vi "Module to Generate Flood of Logs.vi"(7 "Name (\"\" to Use Uuid)":string="CSM-Module") -> ()   [LabVIEW 2017, in "Global Log Handling Capability Example.lvlib"]
doc: "------------- lvcsm -------------\n[CSMStates]\nItem 0 = \"Idle\"\nItem 1 = \"CSM Documentation\"\nItem 2 = \"VI Reference\"\nItem 3 = \"Error Handler\"\nItem 4 = \"Critical Error\"\nItem 5 = \"Target Timeout Error\"\nItem 6 = \"Target Error\"\nItem 7 = \"Async Response\"\nItem 8 = \"Response\"\nItem 9 = \"Async Message Posted\"\nItem 10 = \"Initialize Core Data\"\nItem 11 = \"Exit\"\nItem 12 = \"Data: Initialize\"\nItem 13 = \"Data: Update Indicators\"\nItem 14 = \"Data: Cleanup\"\nItem 15 = \"Macro: Initialize\"\nItem 16 = \"Macro: Exit\"\nItem 17 = \"API: API1\"\nItem 18 = \"API: API2\"\nItem 19 = \"Action: Start\"\nItem 20 = \"Action: action2\"\n\n[CSMStatus]\nItem 0 = \"Error Occurred@Error Handler\""
uses:
  Global Log Handling Capability Example.lvlib
  user.lib/_NEVSTOP/Communicable State Machine(CSM)/AdvanceAPI/CSM - Revert Arguments-Safe String.vi
  user.lib/_NEVSTOP/Communicable State Machine(CSM)/AdvanceAPI/CSM - Make String Arguments Safe.vi
  user.lib/_NEVSTOP/Communicable State Machine(CSM)/AdvanceAPI/CSM - Break Down Multiple States String.vi
  user.lib/_NEVSTOP/Communicable State Machine(CSM)/AdvanceAPI/CSM - Compact Multiple States.vi
  user.lib/_NEVSTOP/Communicable State Machine(CSM)/AdvanceAPI/CSM - Keywords.vi
  user.lib/_NEVSTOP/Communicable State Machine(CSM)/_Shared/Trim Single-line Text.vi
  user.lib/_NEVSTOP/Communicable State Machine(CSM)/Communicable State Machine.lvlib
  user.lib/_NEVSTOP/Communicable State Machine(CSM)/addons/Loop-Support/CSM Loop Support.lvlib
panel:
  in  "Exit":bool
  out "Error Occurred":errorcluster
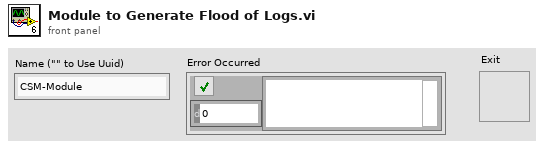
[diagram p1: front panel]
types:
  T1 = enum32{"Invalid", "Standard", "Closed", "Hidden", "Minimized", "Maximized"}
  T2 = enum32{"invalid app kind", "Development System", "Run Time System", "Student Edition", "Embedded LabVIEW", "Evaluation", "Custom"}
  T3 = typedef "Communicable State Machine.lvlib/_CSM_Response Source Message.ctl" = cluster{"‘State":string, "’Arguments":string, "’Error":errorcluster}
  T4 = cluster{"Current VI Reference":refnum<vi>, "Close Panel on Exit?":bool}
  T5 = cluster{"Core":cluster{"Current VI Reference":refnum<vi>, "Close Panel on Exit?":bool}, "Your Boolean data":bool, "Your string data":string}
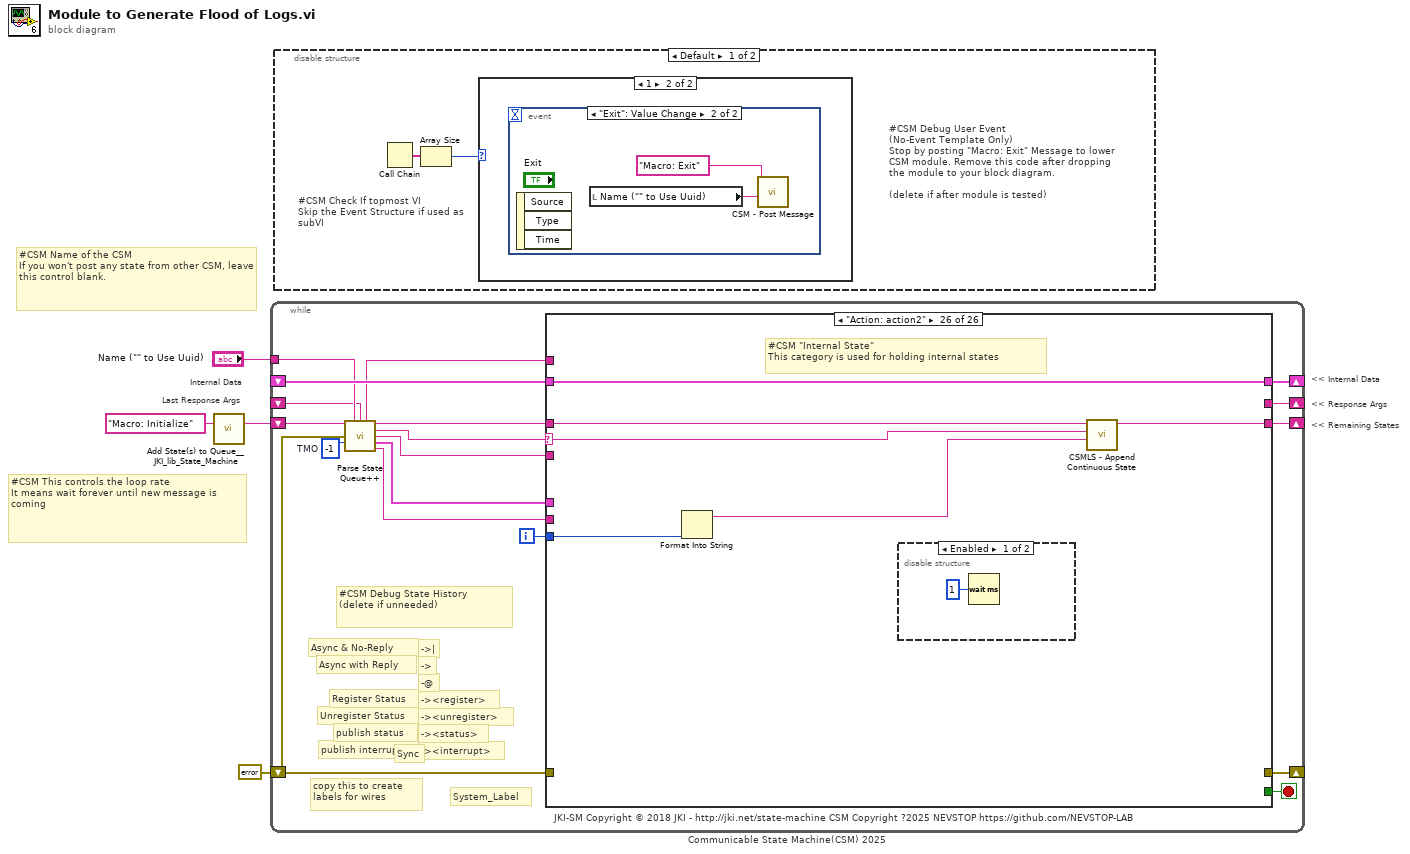
[diagram p0: block diagram]
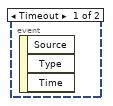
[diagram p3: hidden frame]
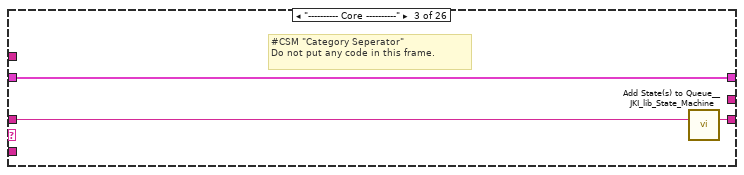
[diagram p7: hidden frame]
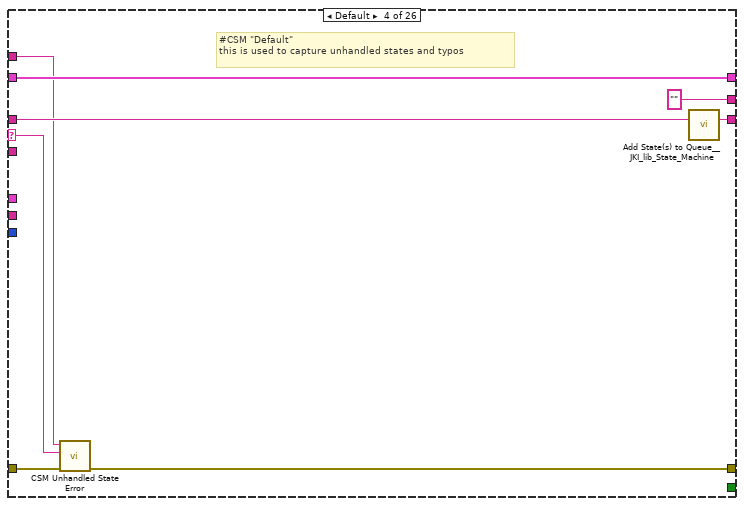
[diagram p8: hidden frame]
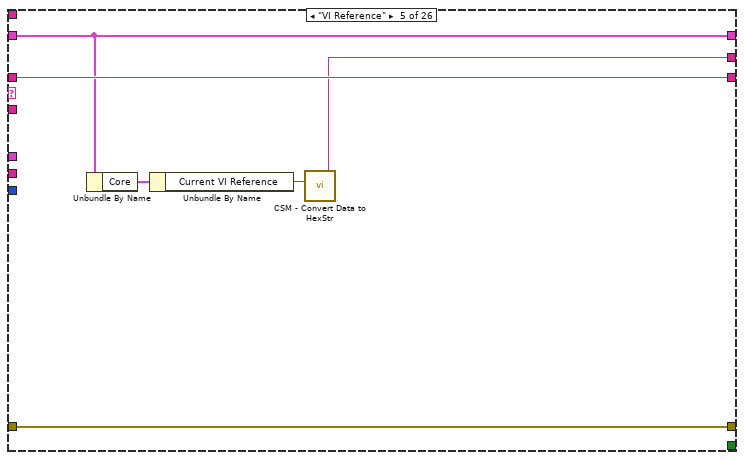
[diagram p9: hidden frame]
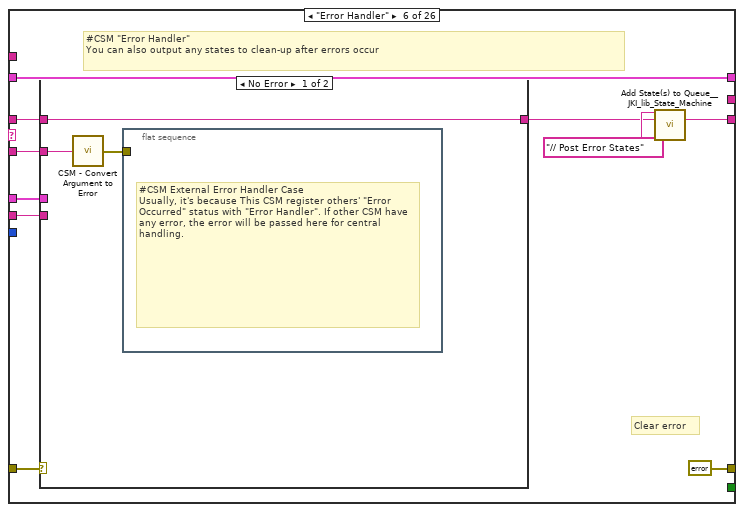
[diagram p10: hidden frame]
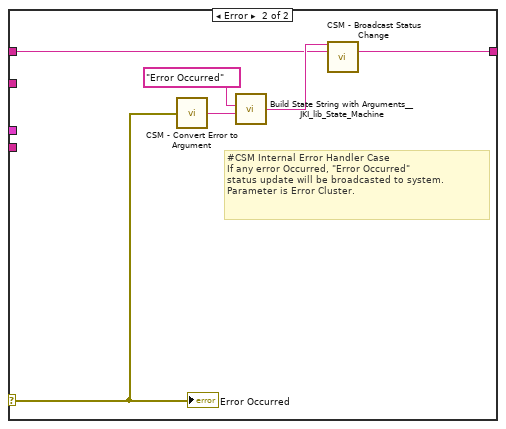
[diagram p11: hidden frame]
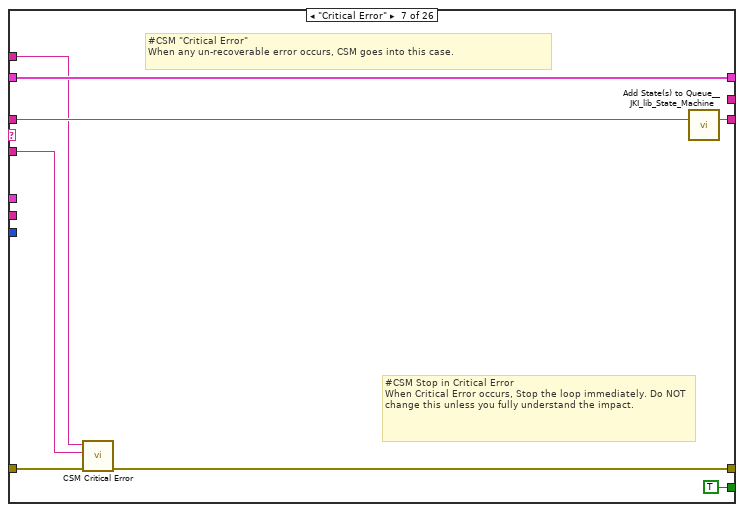
[diagram p12: hidden frame]
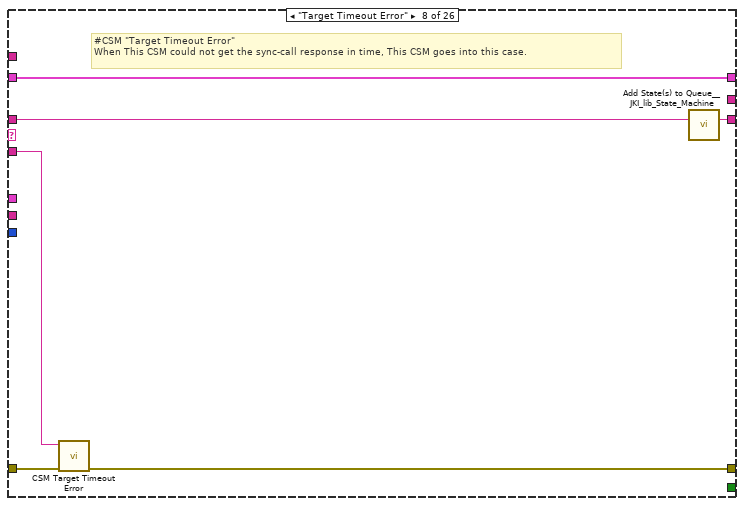
[diagram p13: hidden frame]
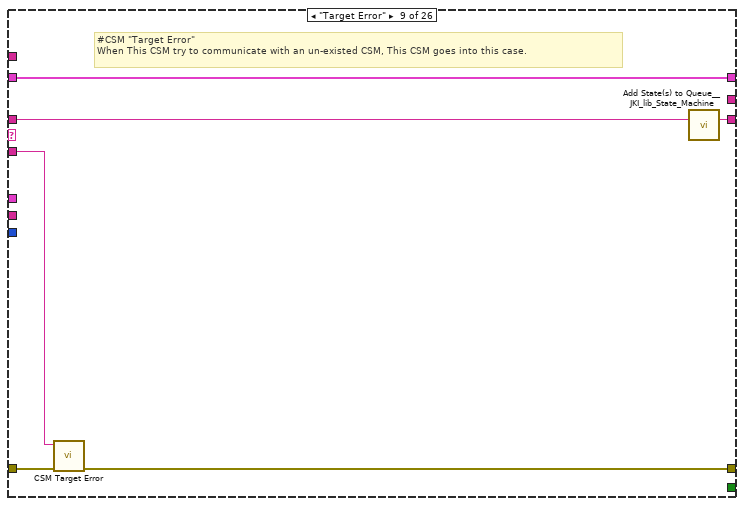
[diagram p14: hidden frame]
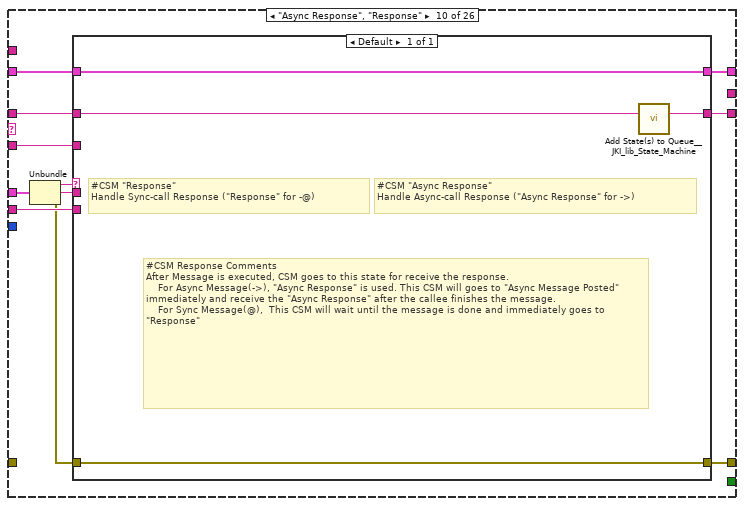
[diagram p15: hidden frame]
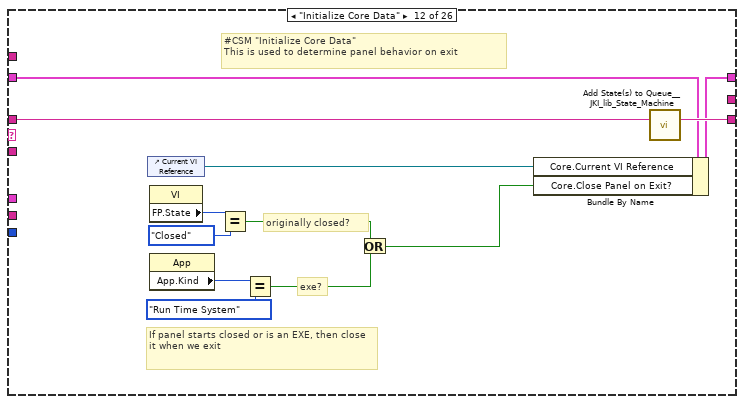
[diagram p17: hidden frame]
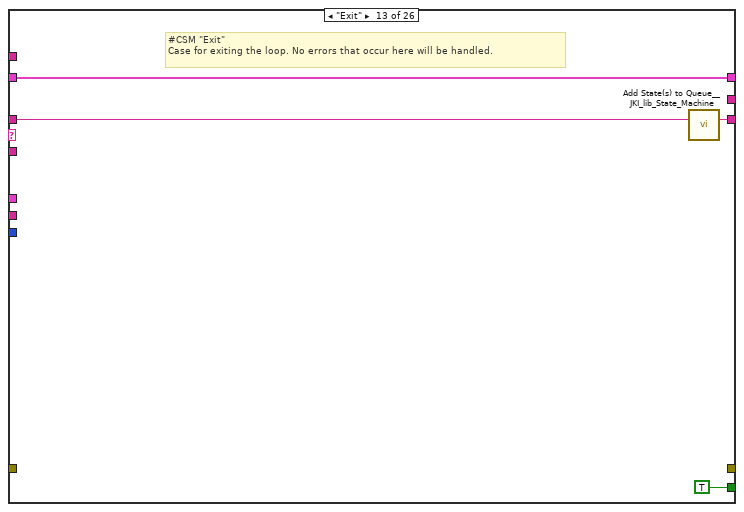
[diagram p18: hidden frame]
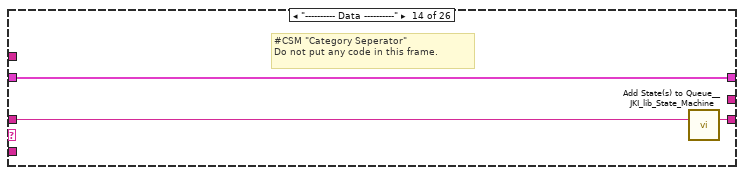
[diagram p19: hidden frame]
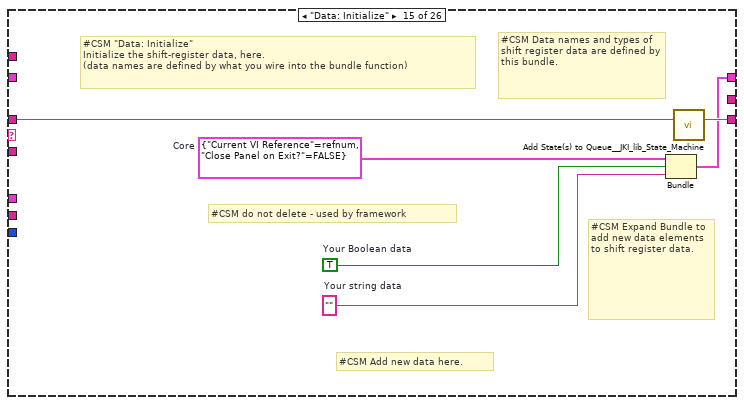
[diagram p20: hidden frame]
diagram:
  # "Last Response Args"
  # "Internal Data"
  # "#CSM Name of the CSM\nIf you won't post any state from other CSM, leave this control blank."
  # "#CSM This controls the loop rate\nIt means wait forever until new message is coming"
  # "<< Internal Data"
  # "<< Response Args"
  # "<< Remaining States"
  n1 = call <vilib>:"Add State(s) to Queue__JKI_lib_State_Machine.vi"("State(s) in (\"\")"="Macro: Initialize" ("Init State(\"Macro: Initialize\")")) -> ("States Out"=w4:string)  [unwired: 14 in]
  n2 = while "Communicable State Machine(CSM) 2025" {
    shift-right: [w17] -> _
    shift-left: _ -> [w16]
    shift-right: [w20] -> _
    shift-left: errorcluster {"status"=FALSE, "code"=0, "source"=""} ("error out") -> [w6]
    shift-right: [w19] -> _
    shift-left: w4 -> [w21]
    tunnel: "Name (\"\" to Use Uuid)" -> [w13]
    shift-right: [w14] -> _
    shift-left: _ -> [w8]
    i -> [w5]
    stop <- w18 stop-if-true
    w15 = -1  # TMO
    # "#CSM Debug State History\n(delete if unneeded)"
    # "-><interrupt>"
    # "-><status>"
    # "-><unregister>"
    # "-><register>"
    # "-@"
    # "->"
    # "->|"
    # "publish interrupt"
    # "publish status"
    # "Unregister Status"
    # "Register Status"
    # "Sync"
    # "Async with Reply"
    # "Async & No-Reply"
    # "JKI-SM Copyright © 2018 JKI - http://jki.net/state-machine CSM Copyright ?2025 NEVSTOP https://github.com/NEVSTOP-LAB"
    # "copy this to create labels for wires"
    # "System_Label"
    n3 = call "Parse State Queue++.vi"("State Queue"=w21, "Name (\"\" to Use UUID)"=w13, "Response Arguments"=w8, "Previous Error"=w6, "Dequeue (1 ms)"=w15) -> ("Name Used"=w7:string, "Remaining States"=w22:string, "Current State"=w9:string, "Arguments"=w10:string, "Additional Information"=w11:T3, "Source CSM"=w12:string)  [unwired: 5 in]
    n4 = case shown="\"Action: action2\"" w9 {
      selector: w9 -> [_ _ _ w33 _ _ _ _ _ _ _ _ _ _ _ _ _ _ _ _ _ _ _ _ _ w166]
      tunnel: w22 -> [w23 w26 w29 w37 w42 w47 w70 w76 w82 w92 w99 w111 w115 w118 w124 w126 w132 w135 w139 w145 w147 w150 w154 w159 w163 w167]
      tunnel: w10 -> [_ _ _ _ _ w46 w66 w73 w79 w86 _ _ _ _ _ _ _ _ _ _ _ _ w152 _ _ _]
      tunnel: w16 -> [w24 w25 w27 w35 w41 w52 w68 w74 w80 w90 w98 w105 w113 w116 _ w125 w127 w133 w137 w143 w146 w149 w153 w157 w161 w168]
      tunnel: [_ _ _ w30 w43 errorcluster {"status"=FALSE, "code"=0, "source"=""} ("error out") w63 w71 w77 w93 _ _ _ _ _ _ w128 _ _ _ _ _ _ _ _ _] -> w20
      tunnel: w6 -> [_ _ _ w31 w43 w50 w64 w72 w78 _ _ _ _ _ _ _ w129 _ _ _ _ _ _ _ _ _]
      tunnel: [w23 w26 w28 w36 w42 w48 w69 w75 w81 w91 w99 w110 w114 w117 w123 w126 w131 w134 w138 w144 w147 w150 w154 w158 w162 w169] -> w19
      tunnel: [_ _ _ _ _ _ TRUE _ _ _ _ _ TRUE _ _ _ _ _ _ _ _ _ _ _ _ _] -> w18
      tunnel: [w24 w25 w27 w35 w41 w52 w68 w74 w80 w89 w98 w109 w113 w116 w122 w125 w127 w133 w137 w143 w146 w149 w153 w157 w161 w168] -> w17
      tunnel: w12 -> [_ _ _ _ _ w45 _ _ _ w87 _ _ _ _ _ _ _ _ _ _ _ _ _ _ _ _]
      tunnel: w11 -> [_ _ _ _ _ w44 _ _ _ w88 _ _ _ _ _ _ _ _ _ _ _ _ _ _ _ _]
      tunnel: [_ _ _ "" w38 _ _ _ _ _ _ _ _ _ _ _ _ _ _ _ _ "API1 Response" w151 _ _ _] -> w14
      tunnel: w7 -> [_ _ _ w32 _ _ w65 _ _ _ _ _ _ _ _ _ _ _ _ _ _ _ _ _ _ _]
      tunnel: w5 -> [_ _ _ _ _ _ _ _ _ _ _ _ _ _ _ _ _ _ _ _ _ _ _ _ _ w165]
      frame "", "Idle" {
        # "#CSM \"Idle/Event Handler\"\nexecutes when the state queue is empty"
      }
      frame "CSM Documentation" {
        # "#CSM State Syntax\n\n// Comment line, all text to the right of “//” will be ignored\n// Local Message Example\nDoSth: DoA >> Arguments\n\n// Sync Call Example\nAPI: xxxx >> Arguments -@ TargetModule\n\n// Async Call Example\nAPI: xxxx >> Arguments -> TargetModule\n\n// Async Call without Reply Example\nAPI: xxxx >> Arguments ->| TargetModule\n\n// Broadcast normal status:\nStatus >> StatusArguments  -><status>\n\n// Broadcast Interrupt status:\nInterrupt >> StatusArguments  -><interrupt>\n\n// Register Source Module's status to Handler Module\nStatus@Source Module >> Handler Module@Handler Module -><register>\n\n// Unegister Source Module's status\nStatus@Source Module >> Handler Module -><unregister>"
        # "#CSM README FIRST\n\nCommunicable State Machine(CSM) is a LabVIEW application framework that builds upon JKI State Machine(JKISM). It follows the pattern of JKISM and extends the keywords to describe message communication between modules, including concepts such as Sync-Message, Async-Message, Subscription/Unsubscription of status - essential elements for creating reusable code modules. For more information, please visit the CSM wiki: https://nevstop-lab.github.io/CSM-Wiki/\n\nFor instructions on JKI State Machine, visit: \n    http://jki.net/state-machine/\nFor information about CSM, visit: \n    https://github.com/NEVSTOP-LAB"
        # "#CSM \"Documentation\"\nCase for holding CSM Documenation"
      }
      frame "---------- Core ----------" {
        # "#CSM \"Category Seperator\"\nDo not put any code in this frame."
        n5 = call <vilib>:"Add State(s) to Queue__JKI_lib_State_Machine.vi"("State(s) in (\"\")"=w29) -> ("States Out"=w28:string)  [unwired: 14 in]
      }
      frame Default {
        # "#CSM \"Default\"\nthis is used to capture unhandled states and typos"
        n6 = call "CSM Unhandled State Error.vi"("error in (no error)"=w31, "Undefined State"=w33, "CSM Name"=w32) -> ("error out"=w30:errorcluster)  [unwired: 8 in]
        n7 = call <vilib>:"Add State(s) to Queue__JKI_lib_State_Machine.vi"("State(s) in (\"\")"=w37) -> ("States Out"=w36:string)  [unwired: 14 in]
      }
      frame "VI Reference" {
        n8 = Unbundle By Name(w41) -> ("Core"=w40:T4)
        n9 = Unbundle By Name(w40) -> ("Current VI Reference"=w39:refnum<vi>)
        n10 = call "CSM - Convert Data to HexStr.vi"("Variant"=w39) -> ("HEX String (0-9,A-F)"=w38:string)  [unwired: 8 in]
      }
      frame "Error Handler" {
        # "#CSM \"Error Handler\"\nYou can also output any states to clean-up after errors occur"
        # "Clear error"
        n11 = case shown="No Error" w50 {
          selector: w50 -> [_ w57]
          tunnel: [w56 w59] -> w49
          tunnel: w47 -> [w56 w58]
          tunnel: w46 -> [w55 _]
          tunnel: w45 -> [_ _]
          tunnel: w44 -> [_ _]
          frame No Error {
            n12 = call "CSM - Convert Argument to Error.vi"("Argument"=w55) -> ("Error"=w54:errorcluster)  [unwired: 4 in]
            n13 = flat-sequence {
              tunnel: w54 -> [_]
              frame #0 {
                # "#CSM External Error Handler Case\nUsually, it's because This CSM register others' \"Error Occurred\" status with \"Error Handler\". If other CSM have any error, the error will be passed here for central handling."
              }
            }
          }
          frame Error {
            # "#CSM Internal Error Handler Case \nIf any error Occurred, \"Error Occurred\" \nstatus update will be broadcasted to system.\nParameter is Error Cluster."
            n14 = call "CSM - Convert Error to Argument.vi"("Error"=w57) -> ("Argument"=w61:string)  [unwired: 4 in]
            n15 = call <vilib>:"Build State String with Arguments__JKI_lib_State_Machine.vi"("Arguments (\"\")"=w61, "State"="Error Occurred" ("Status with Arguments")) -> ("State with Arguments"=w60:string)  [unwired: 4 in]
            n16 = call "CSM - Broadcast Status Change.vi"("Status With Arguments"=w60, "State Queue"=w58) -> ("Remaining States"=w59:string)  [unwired: 13 in]
            "Error Occurred" <- w57
          }
        }
        n17 = call <vilib>:"Add State(s) to Queue__JKI_lib_State_Machine.vi"("State(s) in Front (\"\")"="// Post Error States", "State(s) in (\"\")"=w49) -> ("States Out"=w48:string)  [unwired: 13 in]
      }
      frame "Critical Error" {
        # "#CSM \"Critical Error\"\nWhen any un-recoverable error occurs, CSM goes into this case."
        # "#CSM Stop in Critical Error\nWhen Critical Error occurs, Stop the loop immediately. Do NOT change this unless you fully understand the impact."
        n18 = call "CSM Critical Error.vi"("error in (no error)"=w64, "Arugments (As Reason)"=w66, "CSM Name"=w65) -> ("error out"=w63:errorcluster)  [unwired: 8 in]
        n19 = call <vilib>:"Add State(s) to Queue__JKI_lib_State_Machine.vi"("State(s) in (\"\")"=w70) -> ("States Out"=w69:string)  [unwired: 14 in]
      }
      frame "Target Timeout Error" {
        # "#CSM \"Target Timeout Error\"\nWhen This CSM could not get the sync-call response in time, This CSM goes into this case."
        n20 = call "CSM Target Timeout Error.vi"("error in (no error)"=w72, "Arguments (As CSM Name)"=w73) -> ("error out"=w71:errorcluster)  [unwired: 9 in]
        n21 = call <vilib>:"Add State(s) to Queue__JKI_lib_State_Machine.vi"("State(s) in (\"\")"=w76) -> ("States Out"=w75:string)  [unwired: 14 in]
      }
      frame "Target Error" {
        # "#CSM \"Target Error\"\nWhen This CSM try to communicate with an un-existed CSM, This CSM goes into this case."
        n22 = call "CSM Target Error.vi"("error in (no error)"=w78, "Arguments (As CSM Name)"=w79) -> ("error out"=w77:errorcluster)  [unwired: 9 in]
        n23 = call <vilib>:"Add State(s) to Queue__JKI_lib_State_Machine.vi"("State(s) in (\"\")"=w82) -> ("States Out"=w81:string)  [unwired: 14 in]
      }
      frame "Async Response", "Response" {
        n24 = Unbundle(w88) -> ("‘State"=w85:string, "’Arguments"=w84:string, "’Error"=w83:errorcluster)
        n25 = case shown="Default" w85 {
          tunnel: [w94] -> w91
          tunnel: w92 -> [w95]
          tunnel: [w97] -> w89
          tunnel: w90 -> [w97]
          tunnel: [w96] -> w93
          tunnel: w83 -> [w96]
          tunnel: w87 -> [_]
          tunnel: w86 -> [_]
          tunnel: w84 -> [_]
          frame Default {
            # "#CSM \"Async Response\"\nHandle Async-call Response (\"Async Response\" for ->)"
            # "#CSM \"Response\"\nHandle Sync-call Response (\"Response\" for -@)"
            # "#CSM Response Comments\nAfter Message is executed, CSM goes to this state for receive the response.\n    For Async Message(->), \"Async Response\" is used. This CSM will goes to \"Async Message Posted\" immediately and receive the \"Async Response\" after the callee finishes the message.\n    For Sync Message(@),  This CSM will wait until the message is done and immediately goes to \"Response\""
            n26 = call <vilib>:"Add State(s) to Queue__JKI_lib_State_Machine.vi"("State(s) in (\"\")"=w95) -> ("States Out"=w94:string)  [unwired: 14 in]
          }
        }
      }
      frame "Async Message Posted" {
        # "#CSM \"Async Message Posted\"\nAfter Async Message is posted (-> or ->| ), CSM goes to this state for post-action.\nYou can use Argument - State to tell which Async Message is called."
      }
      frame "Initialize Core Data" {
        # "#CSM \"Initialize Core Data\"\nThis is used to determine panel behavior on exit"
        # "originally closed?"
        # "exe?"
        # "If panel starts closed or is an EXE, then close it when we exit"
        n27 = control-ref of="Current VI Reference"() -> (w103:refnum<vi>)
        n28 = property class="VI"() -> ("FP.State"=w102:T1)  [unwired: 2 in, 2 out]
        n29 = property class="App"() -> ("App.Kind"=w108:T2)  [unwired: 2 in, 2 out]
        n30 = Equal?(x=w102, y=T1."Closed" ("Front Panel Window:State")) -> (x = y?=w100:bool)
        n31 = Equal?(x=w108, y=T2."Run Time System" ("Application:Kind")) -> (x = y?=w106:bool)
        n32 = Or(x=w100, y=w106) -> (x .or. y?=w104:bool)
        n33 = Bundle By Name(cluster=w105, "Core.Current VI Reference"=w103, "Core.Close Panel on Exit?"=w104) -> (w109:T5)
        n34 = call <vilib>:"Add State(s) to Queue__JKI_lib_State_Machine.vi"("State(s) in (\"\")"=w111) -> ("States Out"=w110:string)  [unwired: 14 in]
      }
      frame "Exit" {
        # "#CSM \"Exit\"\nCase for exiting the loop. No errors that occur here will be handled."
        n35 = call <vilib>:"Add State(s) to Queue__JKI_lib_State_Machine.vi"("State(s) in (\"\")"=w115) -> ("States Out"=w114:string)  [unwired: 14 in]
      }
      frame "---------- Data ----------" {
        # "#CSM \"Category Seperator\"\nDo not put any code in this frame."
        n36 = call <vilib>:"Add State(s) to Queue__JKI_lib_State_Machine.vi"("State(s) in (\"\")"=w118) -> ("States Out"=w117:string)  [unwired: 14 in]
      }
      frame "Data: Initialize" {
        w119 = T4 {"Current VI Reference"=refnum, "Close Panel on Exit?"=FALSE}  # Core
        w121 = TRUE  # Your Boolean data
        w120 = ""  # Your string data
        # "#CSM \"Data: Initialize\"\nInitialize the shift-register data, here.\n(data names are defined by what you wire into the bundle function)"
        # "#CSM do not delete - used by framework"
        # "#CSM Expand Bundle to add new data elements to shift register data."
        # "#CSM Add new data here."
        # "#CSM Data names and types of shift register data are defined by this bundle."
        n37 = Bundle("Core"=w119, "Your Boolean data"=w121, "Your string data"=w120) -> (w122:T5)  [unwired: 1 in]
        n38 = call <vilib>:"Add State(s) to Queue__JKI_lib_State_Machine.vi"("State(s) in (\"\")"=w124) -> ("States Out"=w123:string)  [unwired: 14 in]
      }
      frame "Data: Update Indicators" {
      }
      frame "Data: Cleanup" {
        # "#CSM \"Data: Cleanup\"\nCleanup any data and references, here.\n(this is called automatically, by the Macro: Exit)"
        n39 = Unbundle By Name(w127) -> ("Core.Current VI Reference"=w130:refnum<vi>)
        n40 = Close Reference(reference=w130, error in (no error)=w129) -> (error out=w128:errorcluster)
        n41 = call <vilib>:"Add State(s) to Queue__JKI_lib_State_Machine.vi"("State(s) in (\"\")"=w132) -> ("States Out"=w131:string)  [unwired: 14 in]
      }
      frame "---------- Macro ----------" {
        # "#CSM \"Category Seperator\"\nDo not put any code in this frame."
        n42 = call <vilib>:"Add State(s) to Queue__JKI_lib_State_Machine.vi"("State(s) in (\"\")"=w135) -> ("States Out"=w134:string)  [unwired: 14 in]
      }
      frame "Macro: Initialize" {
        # "#CSM \"Macro: Initialize\"\nInitialization Macro (This is called once, when the VI starts)"
        n43 = call <vilib>:"Add State(s) to Queue__JKI_lib_State_Machine.vi"("State(s) in Front (\"\")"="Data: Initialize\nInitialize Core Data\nData: Update Indicators\nAction: Start", "State(s) in (\"\")"=w139) -> ("States Out"=w138:string)  [unwired: 13 in]
      }
      frame "Macro: Exit" {
        # "#CSM \"Macro: Exit\"\nExit Macro (This is called once, when the VI exits)"
        n44 = call <vilib>:"Add State(s) to Queue__JKI_lib_State_Machine.vi"("State(s) in Front (\"\")"="//Exit Sub-Modules ", "State(s) at Back (\"\")"="Data: Cleanup\nExit") -> ("States Out"=w141:string)  [unwired: 13 in]
        n45 = call <vilib>:"Add State(s) to Queue__JKI_lib_State_Machine.vi"("State(s) in Front (\"\")"=w141, "State(s) in (\"\")"=w145) -> ("States Out"=w144:string)  [unwired: 13 in]
      }
      frame "---------- API ----------" {
        # "#CSM \"Category Seperator\"\nDo not put any code in this frame."
      }
      frame "API: API1" {
        # "#CSM API Example\nCopy/Rename this case for your own API"
        # "#CSM >> Source CSM >>\nIf you need to tell who triggered this state , use this string. If it's this case itself, this string is \"\"."
        # "#CSM >> Arguments >>\nDeal with the parameter if any"
        # "#CSM Response\nConnect this to return the response of your API"
      }
      frame "API: API2" {
        # "#CSM API Example\nCopy/Rename this case for your own API"
        # "unpack Hex String  to Variant\nif complex parameter is needed."
        n46 = call "CSM - Convert HexStr to Data.vi"("HEX String"=w152) -> ()  [unwired: 7 in, 2 out]
        n47 = disable-structure shown="Disabled" {
          disable-tunnel: [w155 "API2 Response"] -> w151
          frame Disabled {
            # "pack variant to hexstr \nif complex response is needed."
            # "complex Response"
            n48 = call "CSM - Convert Data to HexStr.vi"() -> ("HEX String (0-9,A-F)"=w155:string)  [unwired: 9 in]
          }
          frame Enabled {
          }
        }
      }
      frame "---------- Action ----------" {
        # "#CSM \"Category Seperator\"\nDo not put any code in this frame."
        n49 = call <vilib>:"Add State(s) to Queue__JKI_lib_State_Machine.vi"("State(s) in (\"\")"=w159) -> ("States Out"=w158:string)  [unwired: 14 in]
      }
      frame "Action: Start" {
        # "#CSM \"Internal State\"\nThis category is used for holding internal states"
        n50 = call "CSMLS - Define Loop State(s).vi"("Loop States"="Action: action2 -><loop>" ("States Queue"), "States Queue"=w163) -> ("Remaining States"=w162:string)  [unwired: 13 in]
      }
      frame "Action: action2" {
        # "#CSM \"Internal State\"\nThis category is used for holding internal states"
        n51 = Format Into String(w165) -> (resulting string=w164:string)  [unwired: 3 in, 1 out]
        n52 = disable-structure shown="Enabled" {
          frame Enabled {
            n53 = Wait (ms)(milliseconds to wait=u32 1) -> ()  [unwired: 1 out]
          }
          frame Disabled {
          }
        }
        n54 = call "CSMLS - Append Continuous State.vi"("Continous Arguments (\"\")"=w164, "Continous State"=w166, "States Queue"=w167) -> ("Remaining States"=w169:string)  [unwired: 8 in]
      }
    }
  }
  n55 = disable-structure shown="Default" {
    frame condition #0 (active) {
      # "#CSM Check If topmost VI\nSkip the Event Structure if used as subVI"
      # "#CSM Debug User Event\n(No-Event Template Only)\nStop by posting \"Macro: Exit\" Message to lower CSM module. Remove this code after dropping the module to your block diagram. \n\n(delete if after module is tested)"
      n56 = Call Chain() -> (call chain=w172:string[])
      n57 = Array Size(array=w172) -> (size(s)=w171:i32)
      n58 = case shown="1" w171 {
        frame Default {
        }
        frame 1 {
          n59 = event shown="[1] \"Exit\": Value Change" {
            selector: _ -> [_ _]
            dyn-events: _ -> [_ _]
            timeout: _ -> [_ _]
            event Timeout {
              n60 = event-data() -> ()  [unwired: 1 in, 3 out]
            }
            event "Exit": Value Change {
              n61 = event-data() -> ()  [unwired: 1 in, 3 out]
              n62 = local read "Name (\"\" to Use Uuid)"() -> (w174:string)
              n63 = call "CSM - Post Message.vi"("Target Module"=w174, "State"="Macro: Exit" ("States")) -> ()  [unwired: 9 in, 1 out]
            }
          }
        }
      }
    }
    frame condition #1 {
    }
  }
